vi "Filter 2d.vi"() -> ()   [LabVIEW 2018]
doc: "filter 2d: This example is an example of a two-dimensional filter, which can be used to perform various operations on images, such as blurring, sharpening, edge detection, etc. It is a matrix composed of numerical weights, commonly referred to as a convolutional kernel or filter kernel. In image processing, the filter kernel performs convolution operations with local regions of the image to change the pixel values of the image and achieve different effects."
uses:
  vi.lib/VIRobotics/opencv_yiku/Mat/Mat_8U/Mat_8U.lvclass
  D:/Program Files/company/National Instruments/LabVIEW 2018/vi.lib/addons/VIRobotics/opencv_yiku/Mat/Mat/Mat.lvclass
  vi.lib/VIRobotics/opencv_yiku/Mat/Mat_32F/Mat_32F.lvclass
  vi.lib/VIRobotics/opencv_yiku/Mat/Create_Mat_32F.vi
  vi.lib/VIRobotics/opencv_yiku/Mat/Create_Mat_8U.vi
  vi.lib/VIRobotics/opencv_yiku/Mat/Mat_32F/set_2d_data.vi
  vi.lib/VIRobotics/opencv_yiku/Cap/Cap.lvclass
  vi.lib/VIRobotics/opencv_yiku/opencv_yiku.lvlib
  vi.lib/VIRobotics/opencv_yiku/Mat/Mat/Mat.lvclass
panel:
  out "current kernel":sgl[][](array[numeric])
  in  "kernel Enum":T1(ring)
  out "new pic":picture
  in  "stop":bool
  out "src pic":picture
  # "Overview: Demonstrates how to Blur images with various low pass filters.\nRequirements: Windows.\nInstructions: \n1.Make sure your computer has a camera.\n2.Run the VI"
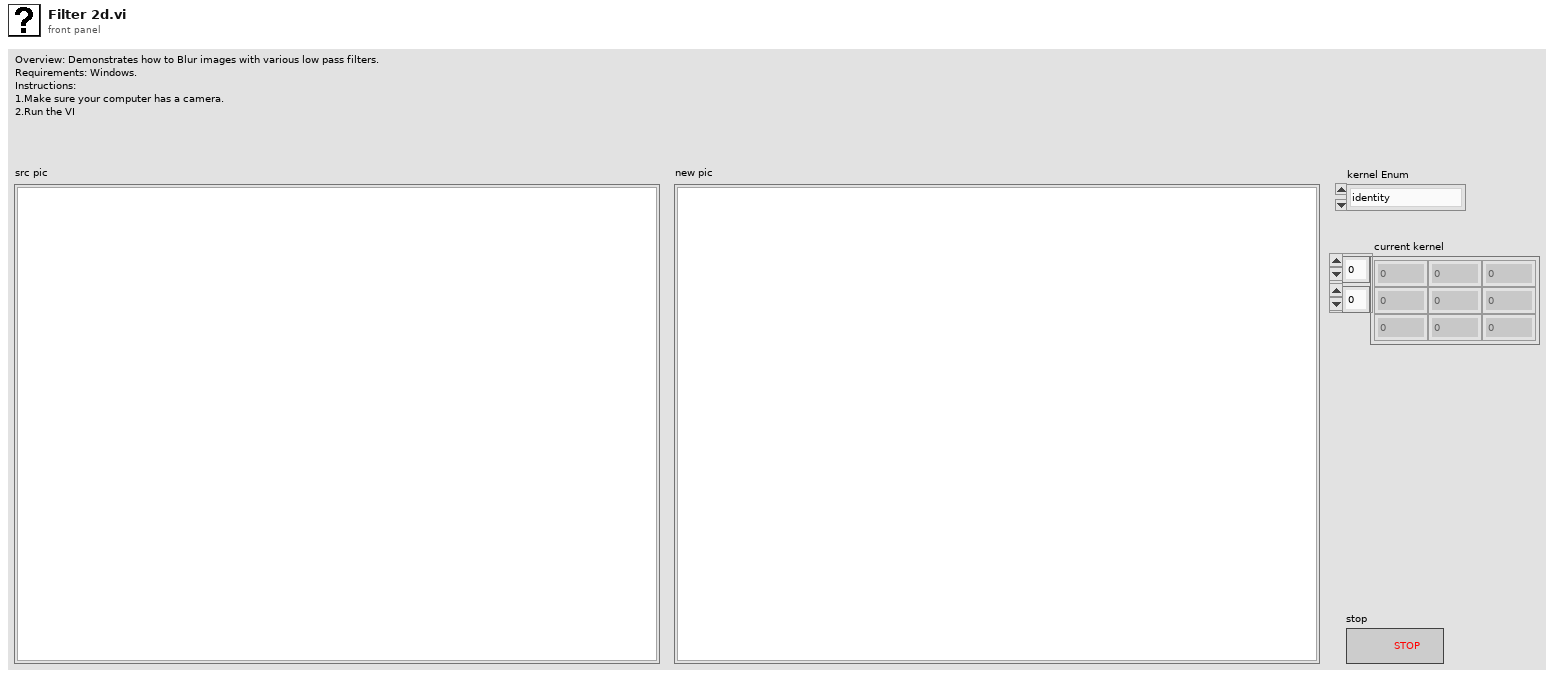
[diagram p1: front panel]
types:
  T1 = enum16{"identity", "outline", "blur", "sobel", "emboss", "sharpen", "laplacian operator"}
  T2 = enum16{"COLOR_BGR2BGRA", "COLOR_BGRA2BGR", "COLOR_BGR2RGBA", "COLOR_RGBA2BGR", "COLOR_BGR2RGB", "COLOR_BGRA2RGBA", "COLOR_BGR2GRAY", "COLOR_RGB2GRAY", "COLOR_GRAY2BGR", "COLOR_GRAY2BGRA"}
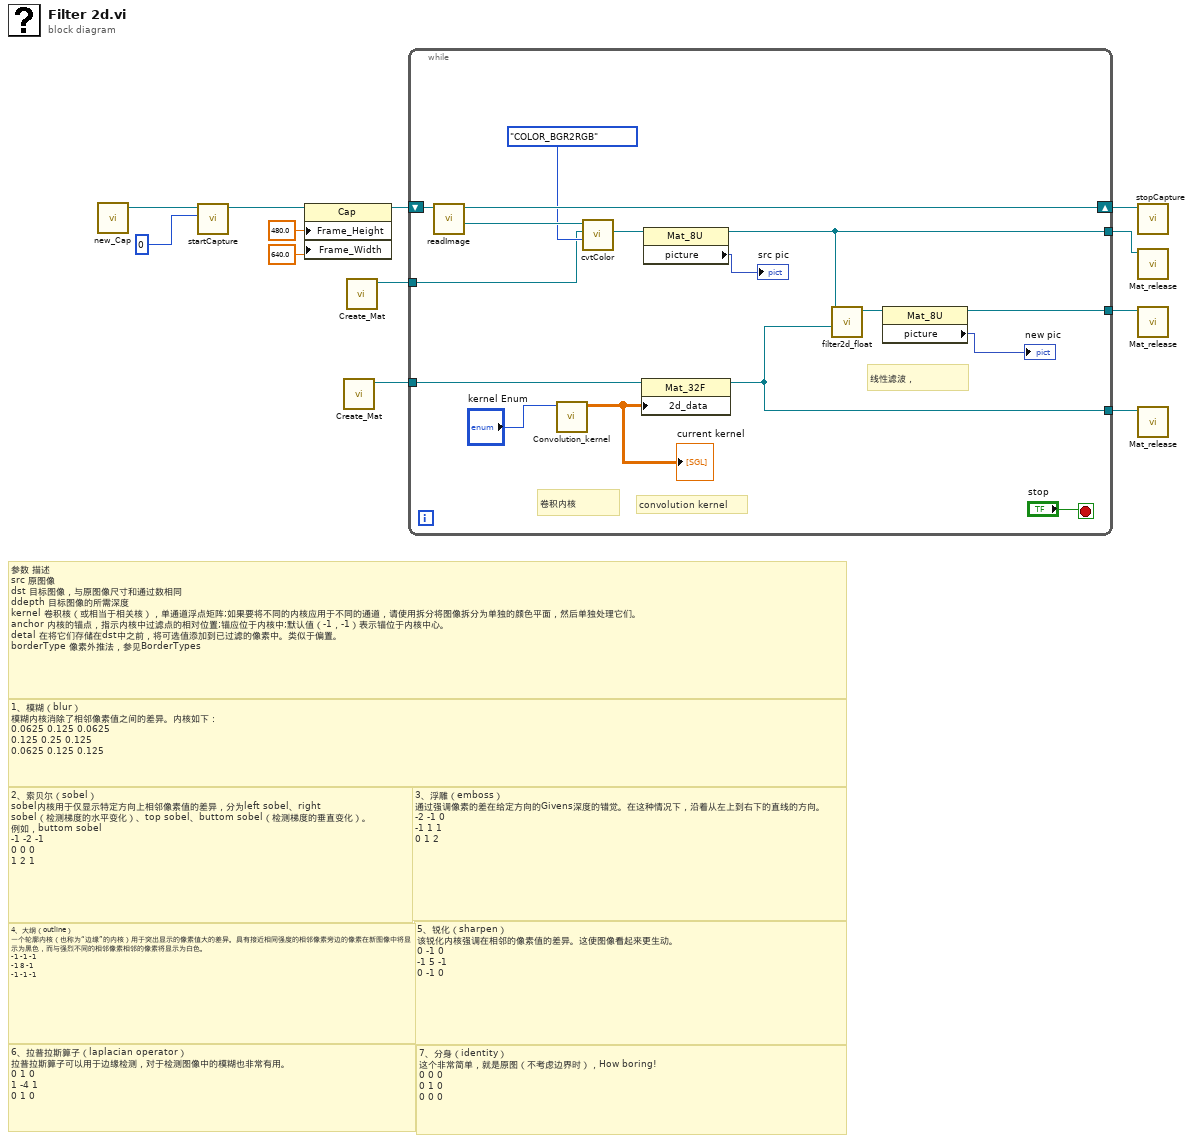
[diagram p0: block diagram]
diagram:
  # "7、分身（identity）\n这个非常简单，就是原图（不考虑边界时），How boring!\n0\t0\t0\n0\t1\t0\n0\t0\t0"
  # "6、拉普拉斯算子（laplacian operator）\n拉普拉斯算子可以用于边缘检测，对于检测图像中的模糊也非常有用。\n0\t1\t0\n1\t-4\t1\n0\t1\t0"
  # "5、锐化（sharpen）\n该锐化内核强调在相邻的像素值的差异。这使图像看起来更生动。\n0\t-1\t0\n-1\t5\t-1\n0\t-1\t0"
  # "4、大纲（outline）\n一个轮廓内核（也称为“边缘”的内核）用于突出显示的像素值大的差异。具有接近相同强度的相邻像素旁边的像素在新图像中将显示为黑色，而与强烈不同的相邻像素相邻的像素将显示为白色。\n-1\t-1\t-1\n-1\t8\t-1\n-1\t-1\t-1"
  # "3、浮雕（emboss）\n通过强调像素的差在给定方向的Givens深度的错觉。在这种情况下，沿着从左上到右下的直线的方向。\n-2\t-1\t0\n-1\t1\t1\n0\t1\t2"
  # "2、索贝尔（sobel）\nsobel内核用于仅显示特定方向上相邻像素值的差异，分为left sobel、right sobel（检测梯度的水平变化）、top sobel、buttom sobel（检测梯度的垂直变化）。\n例如，buttom sobel\n-1\t-2\t-1\n0\t0\t0\n1\t2\t1"
  # "1、模糊（blur）\n模糊内核消除了相邻像素值之间的差异。内核如下：\n0.0625\t0.125\t0.0625\n0.125\t0.25\t0.125\n0.0625\t0.125\t0.125"
  # "参数\t描述\nsrc\t原图像\ndst\t目标图像，与原图像尺寸和通过数相同\nddepth\t目标图像的所需深度\nkernel\t卷积核（或相当于相关核），单通道浮点矩阵;如果要将不同的内核应用于不同的通道，请使用拆分将图像拆分为单独的颜色平面，然后单独处理它们。\nanchor\t内核的锚点，指示内核中过滤点的相对位置;锚应位于内核中;默认值（-1，-1）表示锚位于内核中心。\ndetal\t在将它们存储在dst中之前，将可选值添加到已过滤的像素中。类似于偏置。\nborderType\t像素外推法，参见BorderTypes"
  n1 = call "new_Cap.vi"() -> ("Cap out"=w12:refnum<class "Cap.lvclass">)  [unwired: 10 in, 1 out]
  n2 = call "startCapture.vi"("cameraID"=0, "Cap in"=w12) -> ("Cap out"=w9:refnum<class "Cap.lvclass">)  [unwired: 8 in, 1 out]
  n3 = property class="Cap"(reference=w9, "Frame_Height"=480.0, "Frame_Width"=640.0) -> (reference out=w8:refnum<class "Cap.lvclass">)  [unwired: 1 in, 1 out]
  n4 = call-poly "Create_Mat.vi"() -> ("Mat_32F_out"=w4:refnum<class "Mat_32F.lvclass">)  [unwired: 10 in, 1 out]
  n5 = call-poly "Create_Mat.vi"() -> ("Mat_8U_out"=w1:refnum<class "Mat_8U.lvclass">)  [unwired: 10 in, 1 out]
  n6 = while {
    shift-right: [w27] -> w10
    shift-left: w8 -> [w28]
    tunnel: [w24] -> w5
    tunnel: w4 -> [w21]
    tunnel: [w20] -> w3
    tunnel: [w14] -> w2
    tunnel: w1 -> [w13]
    stop <- "stop" stop-if-true
    # "convolution kernel"
    # "卷积内核"
    # "线性滤波，"
    n7 = call "readImage.vi"("Cap in"=w28) -> ("Mat out"=w25:refnum<class "Mat_8U.lvclass">, "Cap out"=w27:refnum<class "Cap.lvclass">)  [unwired: 8 in, 1 out]
    n8 = call "Convolution_kernel.vi"("kernel Enum"="kernel Enum") -> ("laplacian operator"=w19:sgl[][])  [unwired: 10 in]
    "current kernel" <- w19
    n9 = call "cvtColor.vi"("dstCn"=T2."COLOR_BGR2RGB", "dst"=w13, "src"=w25) -> ("dst out"=w17:refnum<class "Mat_8U.lvclass">)  [unwired: 6 in, 2 out]
    n10 = property class="Mat_32F"(reference=w21, "2d_data"=w19) -> (reference out=w20:refnum<class "Mat_32F.lvclass">)  [unwired: 1 in, 1 out]
    n11 = property class="Mat_8U"(reference=w17) -> (reference out=w14:refnum<class "Mat_8U.lvclass">, "picture"=→"src pic":picture)  [unwired: 1 in, 1 out]
    n12 = call "filter2d_float.vi"("kenerel"=w20, "Mat in"=w14) -> ("dst out"=w22:refnum<class "Mat_8U.lvclass">)  [unwired: 8 in, 1 out]
    n13 = property class="Mat_8U"(reference=w22) -> (reference out=w24:refnum<class "Mat_8U.lvclass">, "picture"=→"new pic":picture)  [unwired: 1 in, 1 out]
  }
  n14 = call "stopCapture.vi"("Cap in"=w10) -> ()  [unwired: 10 in, 1 out]
  n15 = call "Mat_release.vi"("Mat in"=w2) -> ()  [unwired: 10 in, 1 out]
  n16 = call "Mat_release.vi"("Mat in"=w5) -> ()  [unwired: 10 in, 1 out]
  n17 = call "Mat_release.vi"("Mat in"=w3) -> ()  [unwired: 10 in, 1 out]
